vi "Init Services.vi"(8 "error in (no error)":errorcluster, 11 "Vecto in":refnum<class "Vecto.lvclass">) -> (0 "error out":errorcluster, 3 "Vecto out":refnum<class "Vecto.lvclass">)   [LabVIEW 2020, in "Vecto.lvlib" / "Vecto.lvclass"]
uses:
  Vecto.lvclass
  Vecto.lvclass/Vecto.ctl
  Service Container/Service Container.lvclass
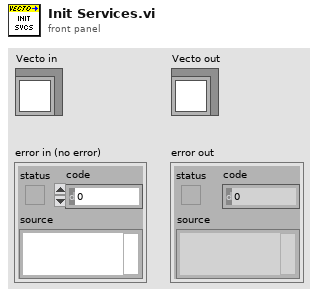
[diagram p1: front panel]
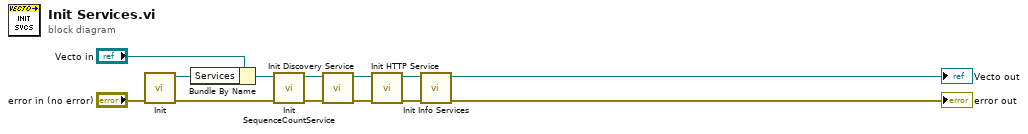
[diagram p0: block diagram]
diagram:
  n1 = call "Init.vi"("error in (no error)"="error in (no error)") -> ("error out"=w8:errorcluster, "Service Container out"=w11:refnum<class "Service Container.lvclass">)  [unwired: 9 in]
  n2 = Bundle By Name(cluster="Vecto in", "Services"=w11) -> (w2:refnum<class "Vecto.lvclass">)
  n3 = call "Init SequenceCountService.vi"("error in (no error)"=w8, "Vecto in"=w2) -> ("error out"=w3:errorcluster, "Vecto out"=w1:refnum<class "Vecto.lvclass">)  [unwired: 8 in]
  n4 = call "Init Discovery Service.vi"("error in (no error)"=w3, "Vecto in"=w1) -> ("error out"=w6:errorcluster, "Vecto out"=w7:refnum<class "Vecto.lvclass">)  [unwired: 8 in]
  n5 = call "Init HTTP Service.vi"("error in (no error)"=w6, "Vecto in"=w7) -> ("error out"=w10:errorcluster, "Vecto out"=w9:refnum<class "Vecto.lvclass">)  [unwired: 8 in]
  n6 = call "Init Info Services.vi"("error in (no error)"=w10, "Vecto in"=w9) -> ("error out"=→"error out":errorcluster, "Vecto out"=→"Vecto out":refnum<class "Vecto.lvclass">)  [unwired: 8 in]
